vi "Remove_Icon_File.vi"(0 "Files In":path[](array[path])) -> (1 "Files Out":path[](array[path]), 2 "Icon files found?":bool)   [LabVIEW 2010]
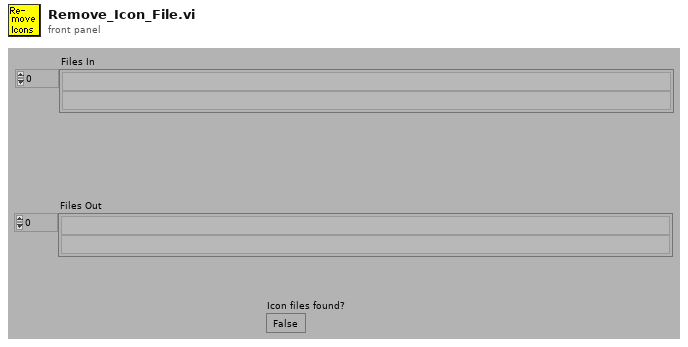
[diagram p1: front panel]
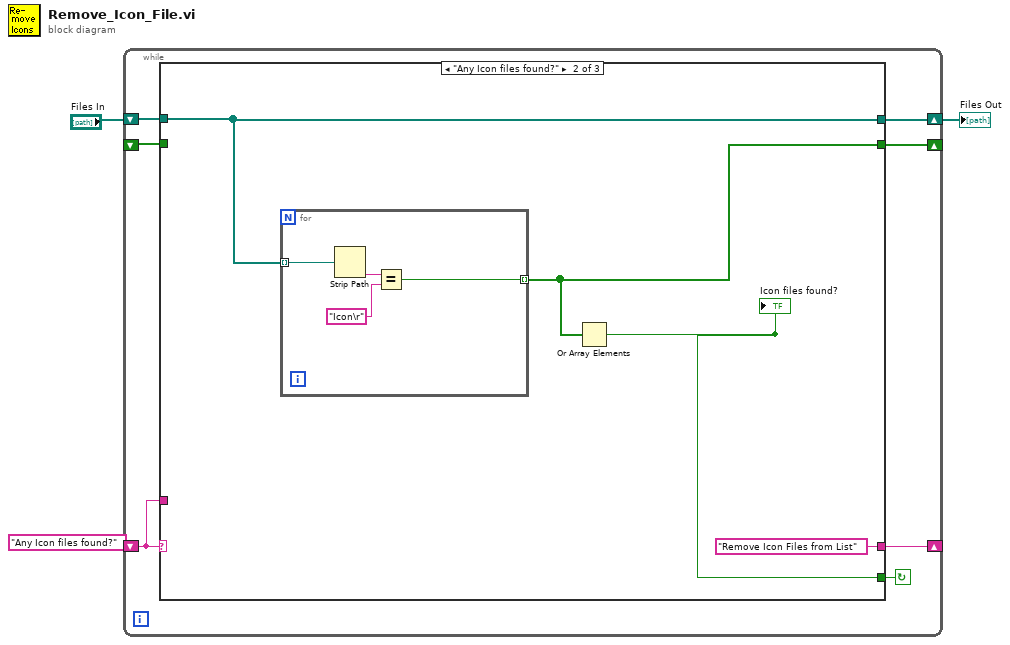
[diagram p0: block diagram]
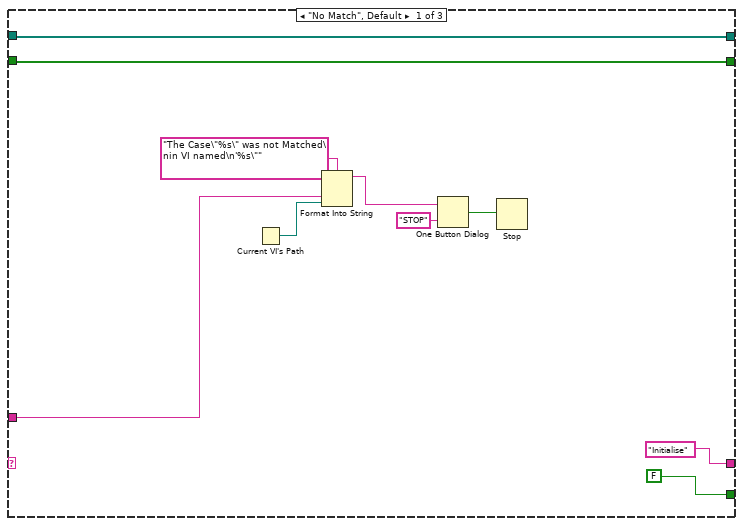
[diagram p2: hidden frame]
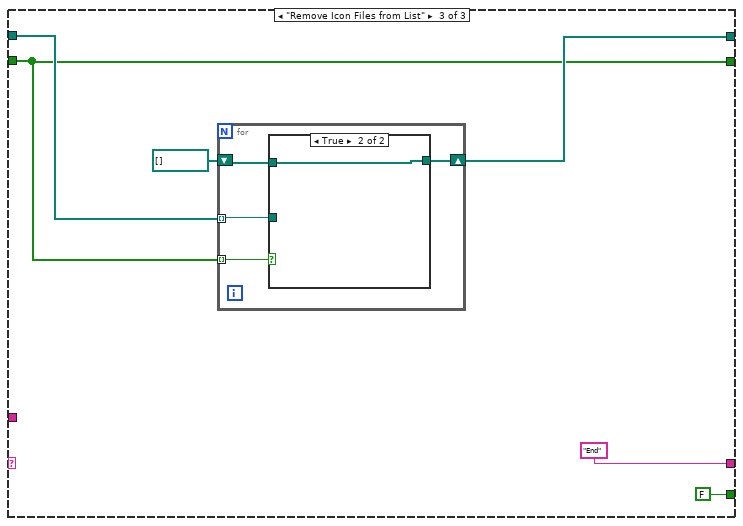
[diagram p3: hidden frame]
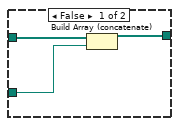
[diagram p4: hidden frame]
diagram:
  n1 = while {
    shift-left: _ -> [w5]
    shift-right: [w6] -> _
    shift-left: "Files In" -> [w7]
    shift-right: [w4] -> w1
    shift-left: "Any Icon files found?" -> [w8]
    shift-right: [w9] -> _
    stop <- w10 continue-if-true
    n2 = case shown="\"Any Icon files found?\"" w8 {
      tunnel: [FALSE w22 FALSE] -> w10
      tunnel: ["Initialise" "Remove Icon Files from List" "End"] -> w9
      tunnel: w8 -> [w15 _ _]
      tunnel: w7 -> [w12 w21 w33]
      tunnel: [w11 w23 w29] -> w6
      tunnel: w5 -> [w11 _ w29]
      tunnel: [w12 w21 w31] -> w4
      frame "No Match", Default {
        n3 = Current VI's Path() -> (path=w14:path)
        n4 = Format Into String(format string="The Case\"%s\" was not Matched\nin VI named\n'%s\"" ("Format String"), w15, w14) -> (resulting string=w18:string)  [unwired: 2 in, 1 out]
        n5 = One Button Dialog(message=w18, button name ("OK")="STOP") -> (true=w16:bool)
        n6 = Stop(stop? (T)=w16) -> ()
      }
      frame "Any Icon files found?" {
        n7 = for {
          tunnel: w21 -> [w28] mode=indexing
          tunnel: [w25] -> w23 mode=indexing
          n8 = Strip Path(path=w28) -> (name=w27:string)  [unwired: 1 out]
          n9 = Equal?(x=w27, y="Icon\r") -> (x = y?=w25:bool)
        }
        n10 = Or Array Elements(Boolean array=w23) -> (logical OR=w22:bool)
        "Icon files found?" <- w22
      }
      frame "Remove Icon Files from List" {
        n11 = for {
          tunnel: w33 -> [w36] mode=indexing
          shift-right: [w35] -> w31
          shift-left: path[] [] -> [w37]
          tunnel: w29 -> [w38] mode=indexing
          n12 = case shown="True" w38 {
            tunnel: w37 -> [w41 w42]
            tunnel: w36 -> [w40 _]
            tunnel: [w39 w42] -> w35
            frame False {
              n13 = Build Array (concatenate)(w41, w40) -> (w39:path[])
            }
            frame True {
            }
          }
        }
      }
    }
  }
  "Files Out" <- w1
